vi "Pid.vi"(0 "Boolean":bool, 11 "Drive Metrics":T1) -> (8 "Right Motor Output":dbl, 10 "Left Motor Output":dbl)   [LabVIEW 2014]
uses:
  Drive Train Metrics.ctl
  CmdFlag.ctl
  <vilib>/addons/control/pid/pid.llb/PID (DBL).vi
  <vilib>/addons/control/pid/NI_PID_pid.lvlib
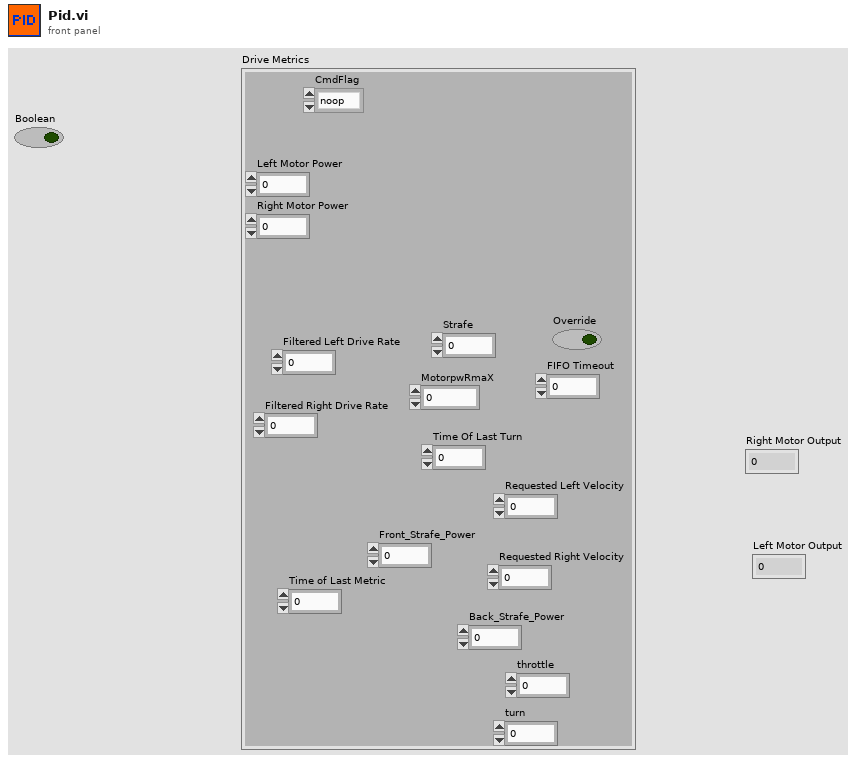
[diagram p1: front panel]
types:
  T1 = typedef "Drive Train Metrics.ctl" = cluster{"CmdFlag":T2, "Right Motor Power":dbl, "Left Motor Power":dbl, "Filtered Left Drive Rate":dbl, "Filtered Right Drive Rate":dbl, "Time of Last Metric":u32, "FIFO Timeout":i32, "Requested Left Velocity":dbl, "Requested Right Velocity":dbl, "throttle":dbl, "turn":dbl, "MotorpwRmaX":i32, "Strafe":dbl, "Override":bool, "Time Of Last Turn":dbl, "Front_Strafe_Power":dbl, "Back_Strafe_Power":dbl}
  T2 = typedef "CmdFlag.ctl" = enum16{"noop", "suspend", "resume"}
  T3 = cluster{"proportional gain (Kc)":dbl, "integral time (Ti, min)":dbl, "derivative time (Td, min)":dbl}
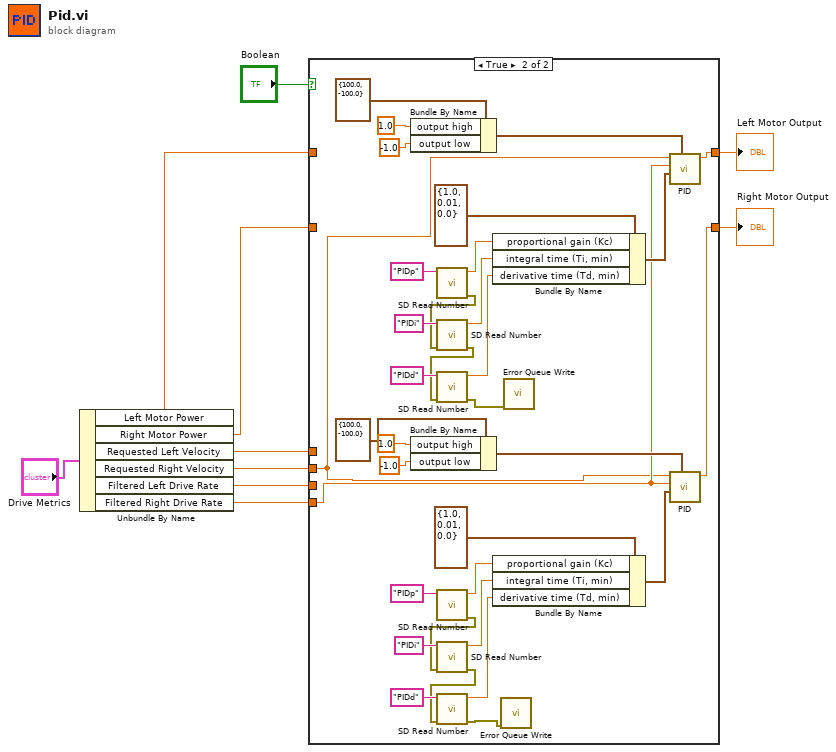
[diagram p0: block diagram]
diagram:
  n1 = Unbundle By Name("Drive Metrics") -> ("Left Motor Power"=w2:dbl, "Right Motor Power"=w1:dbl, "Requested Left Velocity"=w3:dbl, "Requested Right Velocity"=w6:dbl, "Filtered Left Drive Rate"=w4:dbl, "Filtered Right Drive Rate"=w5:dbl)
  n2 = case shown="True" "Boolean" {
    tunnel: w1 -> [w12 _]
    tunnel: [w12 w21] -> w8
    tunnel: w2 -> [w11 _]
    tunnel: [w11 w24] -> w7
    tunnel: w6 -> [_ w19]
    tunnel: w5 -> [_ w20]
    tunnel: w4 -> [_ _]
    tunnel: w3 -> [_ _]
    frame False {
    }
    frame True {
      n3 = Bundle By Name(cluster=cluster{"output high":dbl, "output low":dbl} {"output high"=100.0, "output low"=-100.0} ("output range"), "output high"=1.0, "output low"=-1.0) -> (w33:cluster{"output high":dbl, "output low":dbl})
      n4 = Bundle By Name(cluster=cluster{"output high":dbl, "output low":dbl} {"output high"=100.0, "output low"=-100.0} ("output range"), "output high"=1.0, "output low"=-1.0) -> (w23:cluster{"output high":dbl, "output low":dbl})
      n5 = call <vilib>:"SD Read Number.vi"("Name"="PIDp") -> ("error out"=w18:errorcluster, "Numeric"=w30:dbl)  [unwired: 8 in, 1 out]
      n6 = call <vilib>:"SD Read Number.vi"("error in"=w18, "Name"="PIDi") -> ("error out"=w17:errorcluster, "Numeric"=w29:dbl)  [unwired: 7 in, 1 out]
      n7 = call <vilib>:"SD Read Number.vi"("error in"=w17, "Name"="PIDd") -> ("error out"=w16:errorcluster, "Numeric"=w28:dbl)  [unwired: 7 in, 1 out]
      n8 = call <vilib>:"SD Read Number.vi"("Name"="PIDp") -> ("error out"=w15:errorcluster, "Numeric"=w42:dbl)  [unwired: 8 in, 1 out]
      n9 = call <vilib>:"SD Read Number.vi"("error in"=w15, "Name"="PIDi") -> ("error out"=w14:errorcluster, "Numeric"=w41:dbl)  [unwired: 7 in, 1 out]
      n10 = call <vilib>:"SD Read Number.vi"("error in"=w14, "Name"="PIDd") -> ("error out"=w13:errorcluster, "Numeric"=w40:dbl)  [unwired: 7 in, 1 out]
      n11 = Bundle By Name(cluster=T3 {"proportional gain (Kc)"=1.0, "integral time (Ti, min)"=0.01, "derivative time (Td, min)"=0.0} ("PID gains"), "proportional gain (Kc)"=w30, "integral time (Ti, min)"=w29, "derivative time (Td, min)"=w28) -> (w31:T3)
      n12 = Bundle By Name(cluster=T3 {"proportional gain (Kc)"=1.0, "integral time (Ti, min)"=0.01, "derivative time (Td, min)"=0.0} ("PID gains"), "proportional gain (Kc)"=w42, "integral time (Ti, min)"=w41, "derivative time (Td, min)"=w40) -> (w22:T3)
      n13 = call "Error Queue Write.vi"("error in (no error)"=w13) -> ()  [unwired: 11 in]
      n14 = call "Error Queue Write.vi"("error in (no error)"=w16) -> ()  [unwired: 11 in]
      n15 = call-poly <vilib>:"PID.vi"("output range"=w33, "PID gains"=w31, "process variable"=w20, "setpoint"=w19) -> ("output"=w24:dbl)  [unwired: 6 in, 1 out]
      n16 = call-poly <vilib>:"PID.vi"("output range"=w23, "PID gains"=w22, "process variable"=w20, "setpoint"=w19) -> ("output"=w21:dbl)  [unwired: 6 in, 1 out]
    }
  }
  "Right Motor Output" <- w8
  "Left Motor Output" <- w7
